vi "Switch Data View.vi"(8 "error in (no error)":errorcluster, 10 "Display":enum16{"Waveform", "Table", "Snapshot"}(ring), 11 "Instruments in":refnum<class "Instruments.lvclass">) -> (0 "error out":errorcluster, 3 "Instruments out":refnum<class "Instruments.lvclass">)   [LabVIEW 2023, in "Instruments.lvlib" / "Instruments.lvclass"]
doc: "<b>Switch Data View</b>\nThis method allows a developer to switch displays from waveform, table, and snapshot data. This is a method that's necessary for multiple instruments."
uses:
  Library/Instruments.lvclass
  Library/Instruments.lvclass/Instruments.ctl
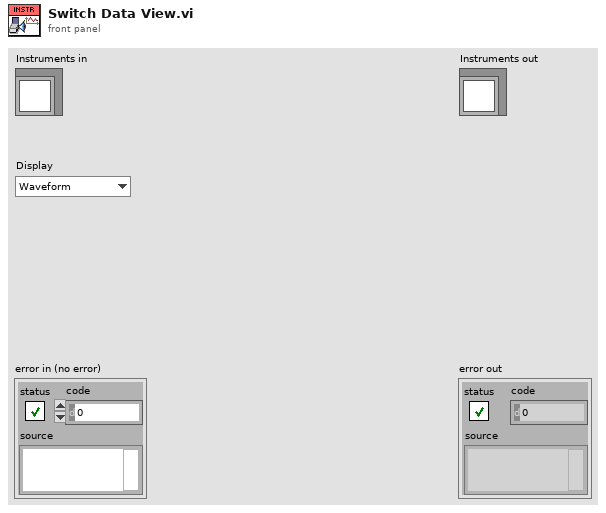
[diagram p1: front panel]
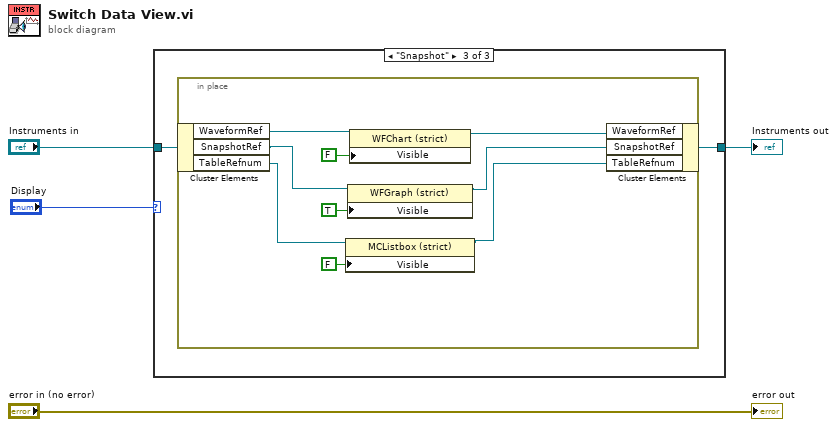
[diagram p0: block diagram]
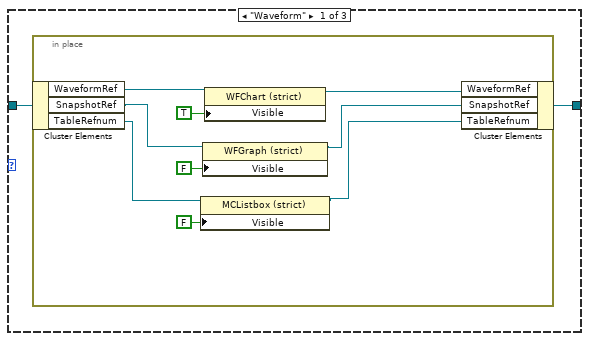
[diagram p2: hidden frame]
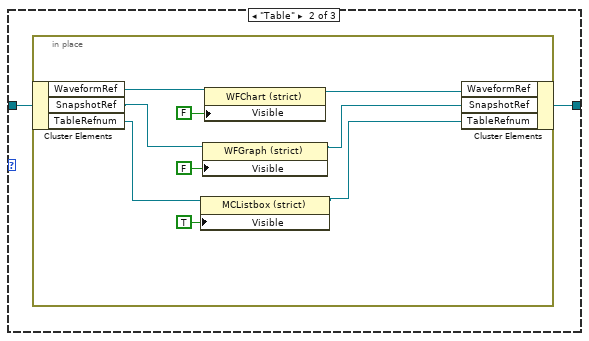
[diagram p3: hidden frame]
diagram:
  n1 = case shown="\"Snapshot\"" "Display" {
    tunnel: "Instruments in" -> [w6 w17 w28]
    tunnel: [w5 w16 w27] -> w3
    frame "Waveform" {
      n2 = in-place {
        n3 = in-place-cluster #1(w6) -> ("WaveformRef"=w15:refnum<vi>, "SnapshotRef"=w13:refnum<vi>, "TableRefnum"=w12:refnum<vi>)
        n4 = property class="MCListbox (strict)"(reference=w12, "Visible"=FALSE) -> (reference out=w10:refnum<vi>)  [unwired: 1 in, 1 out]
        n5 = property class="WFGraph (strict)"(reference=w13, "Visible"=FALSE) -> (reference out=w11:refnum<vi>)  [unwired: 1 in, 1 out]
        n6 = property class="WFChart (strict)"(reference=w15, "Visible"=TRUE) -> (reference out=w14:refnum<vi>)  [unwired: 1 in, 1 out]
        n7 = in-place-cluster #1("WaveformRef"=w14, "SnapshotRef"=w11, "TableRefnum"=w10) -> (w5:refnum<class "Instruments.lvclass">)
      }
    }
    frame "Table" {
      n8 = in-place {
        n9 = in-place-cluster #2(w17) -> ("WaveformRef"=w26:refnum<vi>, "SnapshotRef"=w24:refnum<vi>, "TableRefnum"=w23:refnum<vi>)
        n10 = property class="MCListbox (strict)"(reference=w23, "Visible"=TRUE) -> (reference out=w21:refnum<vi>)  [unwired: 1 in, 1 out]
        n11 = property class="WFGraph (strict)"(reference=w24, "Visible"=FALSE) -> (reference out=w22:refnum<vi>)  [unwired: 1 in, 1 out]
        n12 = property class="WFChart (strict)"(reference=w26, "Visible"=FALSE) -> (reference out=w25:refnum<vi>)  [unwired: 1 in, 1 out]
        n13 = in-place-cluster #2("WaveformRef"=w25, "SnapshotRef"=w22, "TableRefnum"=w21) -> (w16:refnum<class "Instruments.lvclass">)
      }
    }
    frame "Snapshot" {
      n14 = in-place {
        n15 = in-place-cluster #3(w28) -> ("WaveformRef"=w37:refnum<vi>, "SnapshotRef"=w35:refnum<vi>, "TableRefnum"=w34:refnum<vi>)
        n16 = property class="MCListbox (strict)"(reference=w34, "Visible"=FALSE) -> (reference out=w32:refnum<vi>)  [unwired: 1 in, 1 out]
        n17 = property class="WFGraph (strict)"(reference=w35, "Visible"=TRUE) -> (reference out=w33:refnum<vi>)  [unwired: 1 in, 1 out]
        n18 = property class="WFChart (strict)"(reference=w37, "Visible"=FALSE) -> (reference out=w36:refnum<vi>)  [unwired: 1 in, 1 out]
        n19 = in-place-cluster #3("WaveformRef"=w36, "SnapshotRef"=w33, "TableRefnum"=w32) -> (w27:refnum<class "Instruments.lvclass">)
      }
    }
  }
  "Instruments out" <- w3
  "error out" <- "error in (no error)"
